vi "Operate.vi"(8 "error in (no error)":errorcluster, 11 "Divide in":refnum<class "Divide.lvclass">) -> (0 "error out":errorcluster, 3 "Divide out":refnum<class "Divide.lvclass">)   [LabVIEW 2020, in "Divide.lvclass"]
doc: "This methods is used as a child to perform division operation"
uses:
  Divide.lvclass
  D:/labview/Assignment 24/Math Operations/Math Operations.lvclass
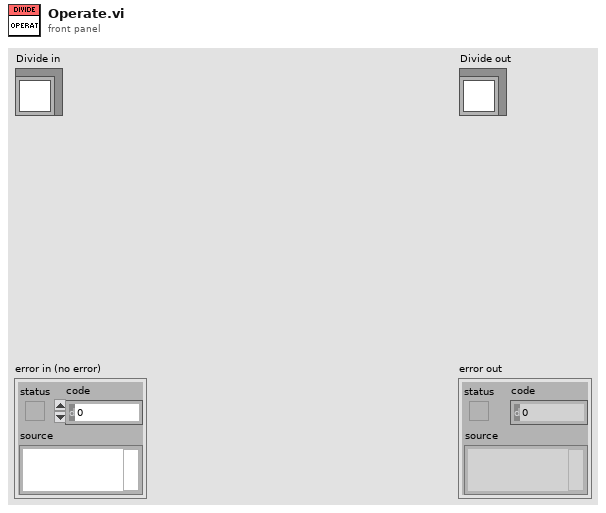
[diagram p1: front panel]
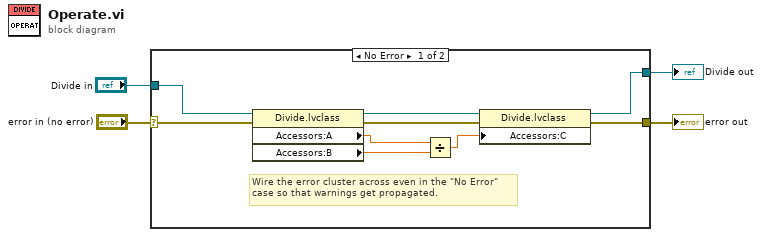
[diagram p0: block diagram]
diagram:
  n1 = case shown="No Error" "error in (no error)" {
    selector: "error in (no error)" -> [w13 w15]
    tunnel: [w5 w15] -> w3
    tunnel: [w6 w14] -> w1
    tunnel: "Divide in" -> [w11 w14]
    frame No Error {
      # "Wire the error cluster across even in the \"No Error\"\ncase so that warnings get propagated."
      n2 = property class="Divide.lvclass"(reference=w11, error in=w13) -> (reference out=w10:refnum<class "Divide.lvclass">, error out=w12:errorcluster, "Accessors:A"=w9:dbl, "Accessors:B"=w8:dbl)
      n3 = Divide(x=w9, y=w8) -> (x/y=w7:dbl)
      n4 = property class="Divide.lvclass"(reference=w10, error in=w12, "Accessors:C"=w7) -> (reference out=w6:refnum<class "Divide.lvclass">, error out=w5:errorcluster)
    }
    frame Error {
    }
  }
  "error out" <- w3
  "Divide out" <- w1
